vi "Read Client ID.vi"(8 "error in (no error)":errorcluster, 11 "Oauth2 in":refnum<class "Oauth2.lvclass">) -> (0 "error out":errorcluster, 2 "Client ID":string, 3 "Oauth2 out":refnum<class "Oauth2.lvclass">)   [LabVIEW 2020, in "Oauth2.lvclass"]
uses:
  Oauth2.lvclass
  Oauth2.lvclass/Oauth2.ctl
  OAuthToken/OAuthAccessToken.lvclass
  OAuthToken/OAuth2 Token Element -- enum.ctl
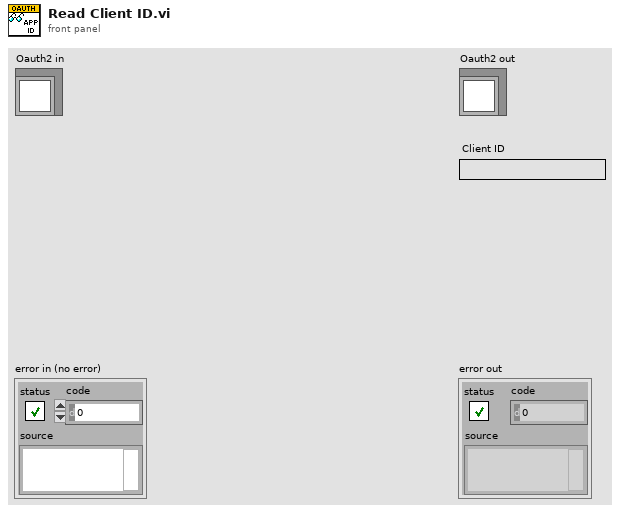
[diagram p1: front panel]
types:
  T1 = typedef "OAuthAccessToken.lvclass/OAuth2 Token Element -- enum.ctl" = enum16{"client_id", "client_secret", "response_type", "scope", "redirect_uri", "error", "error_description", "error_uri", "grant_type", "code", "access_token", "token_type", "expires_in", "username", "password", "refresh_token", "code_challenge", "code_challenge_method", "reverse_proxy_uri", "endpoint element"}
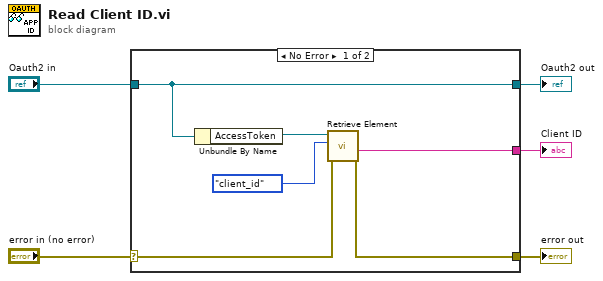
[diagram p0: block diagram]
diagram:
  n1 = case shown="No Error" "error in (no error)" {
    selector: "error in (no error)" -> [w8 w12]
    tunnel: [w7 w12] -> w4
    tunnel: [w11 w13] -> w2
    tunnel: "Oauth2 in" -> [w11 w13]
    tunnel: [w6 _] -> w1
    frame No Error {
      n2 = Unbundle By Name(w11) -> ("AccessToken"=w10:refnum<class "OAuthAccessToken.lvclass">)
      n3 = call "Retrieve Element.vi"("error in (no error)"=w8, "Token element"=OAuth2_Token_Element_--_enum."client_id", "OAuthAccessToken in"=w10) -> ("error out"=w7:errorcluster, "Value"=w6:string)  [unwired: 4 in, 3 out]
    }
    frame Error {
    }
  }
  "error out" <- w4
  "Oauth2 out" <- w2
  "Client ID" <- w1
